vi "SetTilesPng.vi"(5 "DefaultTileCode":u32, 6 "Draw (true)":bool=TRUE, 7 "Tiles":cluster{"Color":fxp<+,3,3>, "TileCode":u32}[](array[cluster]), 8 "error in (no error)":errorcluster, 9 "Position":T1, 10 "Path":path, 11 "Game in":refnum<class "Game.lvclass">) -> (0 "error out":errorcluster, 1 "Tilecodes":u32[][](array[numeric]), 2 "size(tiles)":T1, 3 "Game out":refnum<class "Game.lvclass">)   [LabVIEW 2019, in "RT_Game.lvlib" / "Game.lvclass"]
uses:
  Game.lvclass
  Coordinate.ctl
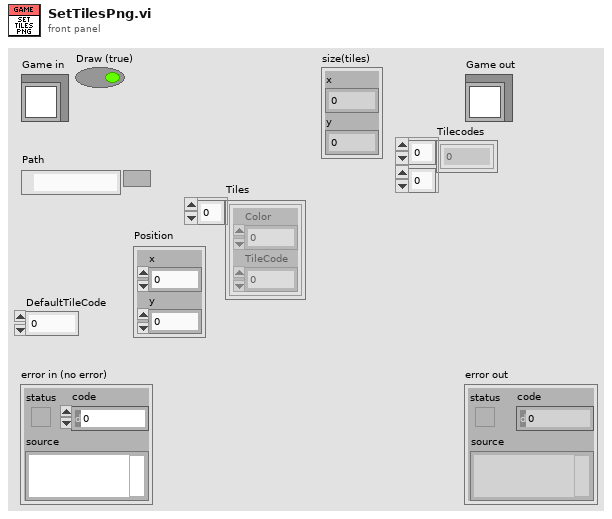
[diagram p1: front panel]
types:
  T1 = typedef "RT_Game.lvlib/Game.lvclass/Coordinate.ctl" = cluster{"x":dbl, "y":dbl}
  T2 = typedef "Color (U64)" = cluster{"Plane 3 (Blue)":u16, "Plane 2 (Green)":u16, "Plane 1 (Red)":u16, "Plane 4 (alpha)":u16}
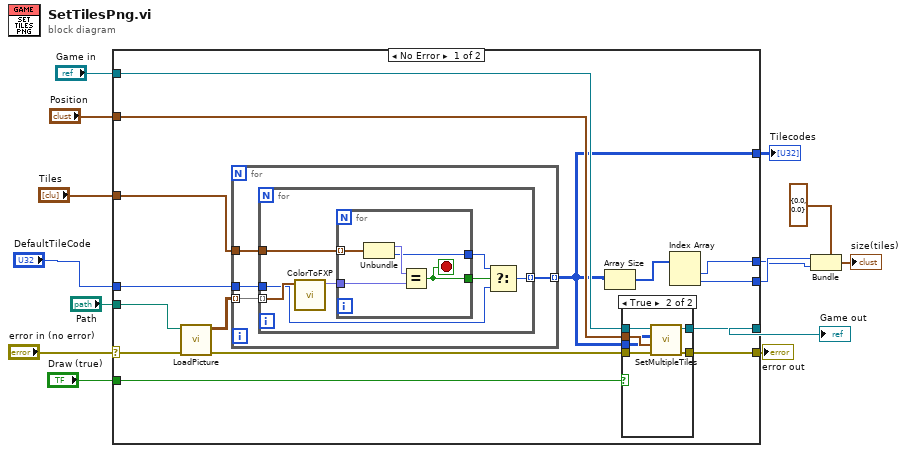
[diagram p0: block diagram]
diagram:
  n1 = case shown="No Error" "error in (no error)" {
    selector: "error in (no error)" -> [w29 w55]
    tunnel: [w25 w55] -> w13
    tunnel: [w24 w54] -> w11
    tunnel: "Game in" -> [w23 w54]
    tunnel: "Path" -> [w27 _]
    tunnel: "DefaultTileCode" -> [w22 _]
    tunnel: "Tiles" -> [w21 _]
    tunnel: "Position" -> [w20 _]
    tunnel: [w18 _] -> w6
    tunnel: [w17 _] -> w7
    tunnel: [w16 _] -> w3
    tunnel: "Draw (true)" -> [w15 _]
    frame No Error {
      n2 = call "LoadPicture.vi"("error in (no error)"=w29, "path to PNG file"=w27) -> ("error out"=w28:errorcluster, "Image Pixels (U64)"=w26:T2[][])  [unwired: 8 in]
      n3 = for {
        tunnel: w26 -> [w41] mode=indexing
        tunnel: w21 -> [w40]
        tunnel: w22 -> [w39]
        tunnel: [w38] -> w16 mode=indexing
        n4 = for {
          tunnel: w41 -> [w48] mode=indexing
          tunnel: w40 -> [w47]
          tunnel: w39 -> [w43]
          tunnel: [w42] -> w38 mode=indexing
          n5 = call "ColorToFXP.vi"("Color (U64)"=w48) -> ("Numeric"=w46:fxp<+,3,3>)  [unwired: 10 in]
          n6 = for {
            tunnel: w47 -> [w53] mode=indexing
            tunnel: w46 -> [w51]
            tunnel: [w50] -> w44
            tunnel: [w49] -> w45
            stop <- w49 stop-if-true
            n7 = Unbundle(w53) -> ("Color"=w52:fxp<+,3,3>, "TileCode"=w50:u32)
            n8 = Equal?(x=w52, y=w51) -> (x = y?=w49:bool)
          }
          n9 = Select(t=w44, s=w45, f=w43) -> (s? t:f=w42:u32)
        }
      }
      n10 = Array Size(array=w16) -> (size(s)=w19:i32[])
      n11 = case shown="True" w15 {
        tunnel: w28 -> [w30 w37]
        tunnel: [w30 w36] -> w25
        tunnel: [w31 w35] -> w24
        tunnel: w23 -> [w31 w34]
        tunnel: w20 -> [_ w33]
        tunnel: w16 -> [_ w32]
        frame False {
        }
        frame True {
          n12 = call "SetMultipleTiles.vi"("error in (no error)"=w37, "Position"=w33, "TileCodes"=w32, "Game in"=w34) -> ("error out"=w36:errorcluster, "Game out"=w35:refnum<class "Game.lvclass">)  [unwired: 6 in]
        }
      }
      n13 = Index Array(array=w19) -> (element #1=w18:i32, element #2=w17:i32)  [unwired: 2 in]
    }
    frame Error {
    }
  }
  "error out" <- w13
  "Game out" <- w11
  "Tilecodes" <- w3
  n14 = Bundle(cluster=T1 {"x"=0.0, "y"=0.0} ("Coordinate"), "x"=w7, "y"=w6) -> (→"size(tiles)":T1)
